vi "VNARP-Detect resonance.vi"(9 "RP VNA SETTING":T1={"F start"=200000, "F stop"=2000500, "Sweep size"=1000, "Decimation"=5000, "F_corr"=0, "Ph_OUT1"=0, "Ph_OUT2"=0, "OUT_Lvl1"=32700, "OUT_Lvl2"=32700, "GPIO"=0}, 10 "VNA DATA CLUSTER":T3 {"Time Stamp Indicator - Long" format="%<%.0X %x>T"}, 11 "RESONNANCE DETECTION":T2 {"Parabolic fit"."Span type" items=["Points N°", "Frequency (Hz)", "Span %"]; "METHOD" items=["Maximum amplitude", "Max on parabolic fit"]}) -> (0 "error out":errorcluster caption="sortie d'erreur", 2 "Resonant frequency":ext, 3 "Parabolic fit":cluster{cluster{dbl, dbl}[]})   [LabVIEW 2021]
uses:
  Spectrum data.ctl
  Resonnance detection.ctl
  vna settings.ctl
panel:
  # "PARAMETERS"
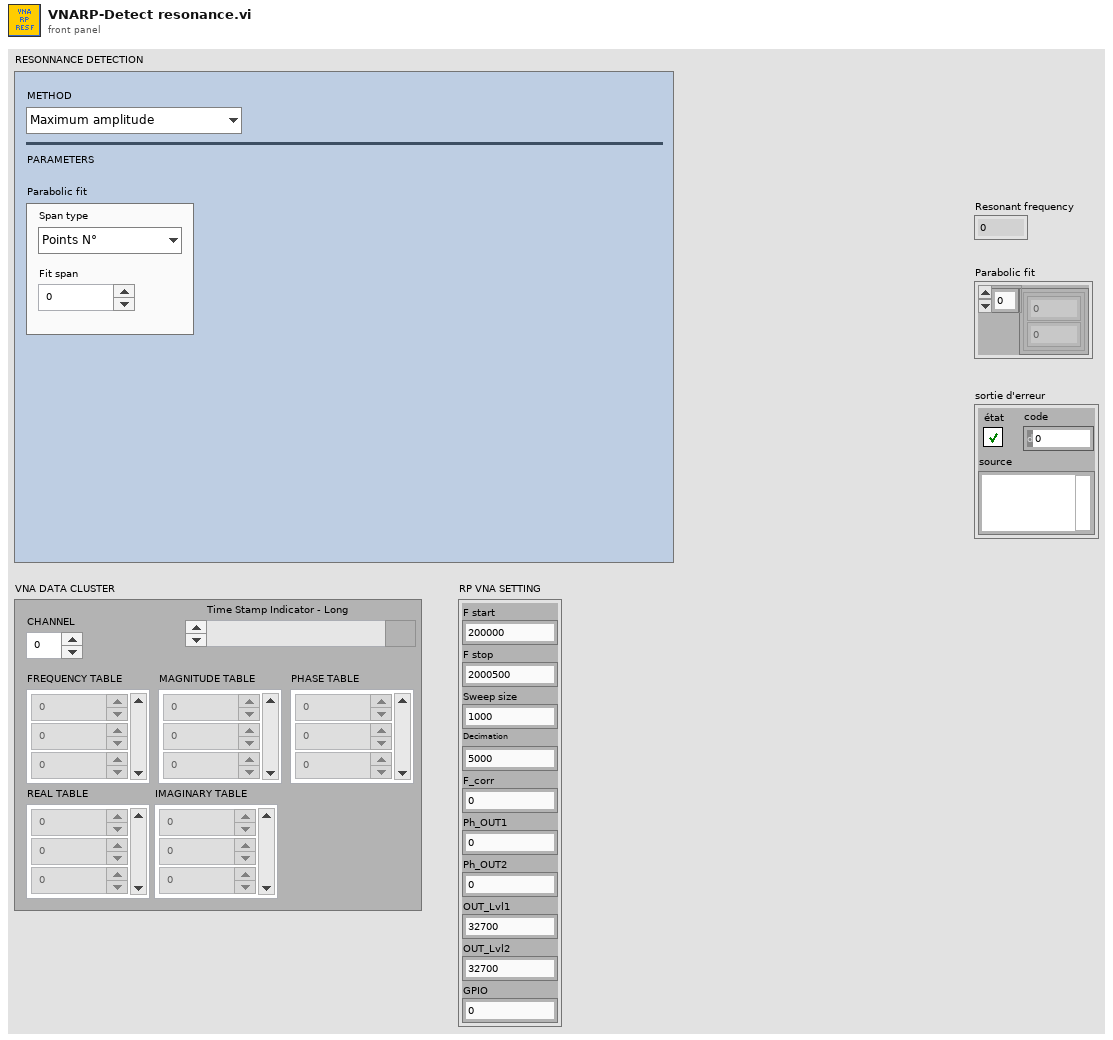
[diagram p1: front panel]
types:
  T1 = typedef "vna settings.ctl" = cluster{"F start":u32, "F stop":u32, "Sweep size":u32, "Decimation":u32, "F_corr":u32, "Ph_OUT1":u32, "Ph_OUT2":u32, "OUT_Lvl1":u32, "OUT_Lvl2":u32, "GPIO":u32}
  T2 = typedef "Resonnance detection.ctl" = cluster{"METHOD":u16, "Parabolic fit":cluster{"Span type":u16, "Fit span":dbl}}
  T3 = typedef "Spectrum data.ctl" = cluster{"CHANNEL":dbl, "FREQUENCY TABLE":ext[], "MAGNITUDE TABLE":ext[], "PHASE TABLE":ext[], "REAL TABLE":ext[], "IMAGINARY TABLE":ext[], "Time Stamp Indicator - Long":timestamp}
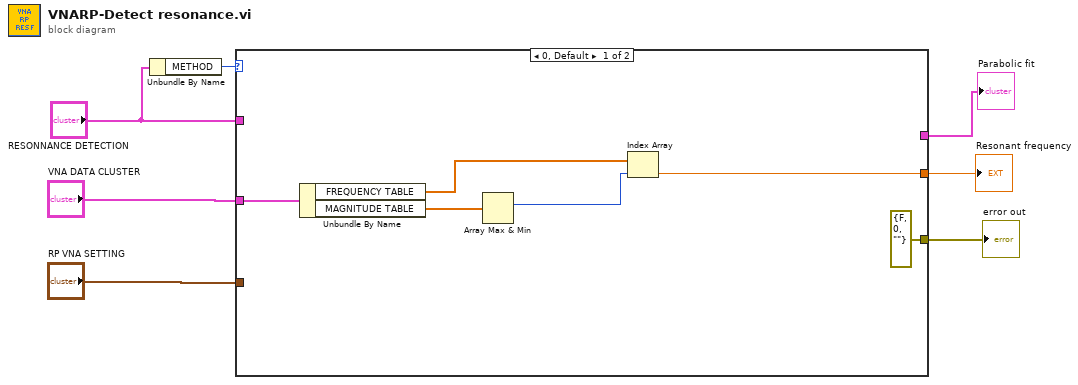
[diagram p0: block diagram]
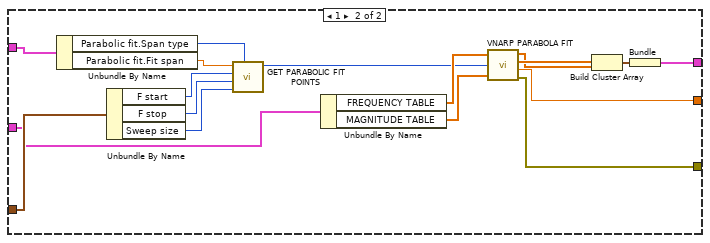
[diagram p2: hidden frame]
diagram:
  n1 = Unbundle By Name("RESONNANCE DETECTION") -> ("METHOD"=w7:u16)
  n2 = case shown="0, Default" w7 {
    tunnel: "VNA DATA CLUSTER" -> [w13 w17]
    tunnel: [w9 w16] -> w6
    tunnel: "RESONNANCE DETECTION" -> [_ w19]
    tunnel: "RP VNA SETTING" -> [_ w18]
    tunnel: [_ w15] -> w2
    tunnel: [errorcluster {"status"=FALSE, "code"=0, "source"=""} ("error out") w14] -> w1
    frame 0, Default {
      n3 = Unbundle By Name(w13) -> ("FREQUENCY TABLE"=w11:ext[], "MAGNITUDE TABLE"=w12:ext[])
      n4 = Array Max & Min(array=w12) -> (max index (indices)=w10:i32)  [unwired: 3 out]
      n5 = Index Array(array=w11, index=w10) -> (element=w9:ext)
    }
    frame 1 {
      n6 = Unbundle By Name(w19) -> ("Parabolic fit.Span type"=w22:u16, "Parabolic fit.Fit span"=w21:dbl)
      n7 = Unbundle By Name(w18) -> ("F start"=w23:u32, "F stop"=w24:u32, "Sweep size"=w25:u32)
      n8 = call "GET PARABOLIC FIT POINTS.vi"("Data entry"=w22, "Sweep size"=w25, "F stop"=w24, "F start"=w23, "Parabolic fit span"=w21) -> ("Points"=w20:i32)  [unwired: 6 in]
      n9 = Unbundle By Name(w17) -> ("FREQUENCY TABLE"=w26:ext[], "MAGNITUDE TABLE"=w27:ext[])
      n10 = call "VNARP PARABOLA FIT.vi"("Freq Table IN"=w26, "Fit length"=w20, "Y IN"=w27) -> ("Best Polynomial Fit"=w29:dbl[], "Fit Span"=w30:dbl[], "Parabol max position"=w16:dbl, "error out"=w14:errorcluster)
      n11 = Build Cluster Array(w30, w29) -> (w28:cluster{dbl, dbl}[])
      n12 = Bundle(w28) -> (w15:cluster{cluster{dbl, dbl}[]})  [unwired: 1 in]
    }
  }
  "Resonant frequency" <- w6
  "Parabolic fit" <- w2
  "error out" <- w1
